vi "ICM Test Program.vi"() -> ()   [LabVIEW 2018]
doc: "Test Program.vi\n\nThis is a simple program that uses the ICM to demonstrate its structure.\n\nInstrument Communication Module Version 1.0\nDecember, 2017 Original Code Consulting David Thomson\n www.originalcode.com"
uses:
  Scaling/Scaling.lvclass
  Scaling/Scaling.lvclass/Scaling.ctl
  Query/Query.lvclass/Query.ctl
  Query/Read Cycle Time (ms).vi
  Initialize/Initialize.lvclass
  Parser/Parser.lvclass
  Output/Output.lvclass
  Query/Query.lvclass
  Bus/Bus.lvclass
panel:
  in  "Controller Values":dbl[](array[numeric])
  out "Enabled Controllers":string[](array[string])
  out "Scaled Values":dbl[](array[numeric])
  in  "stop":bool
  out "Enabled Channels":string[](array[string])
  out "Data Values":dbl[](array[numeric])
  out "String Read":string
  out "error out":errorcluster
  out "Config File":path
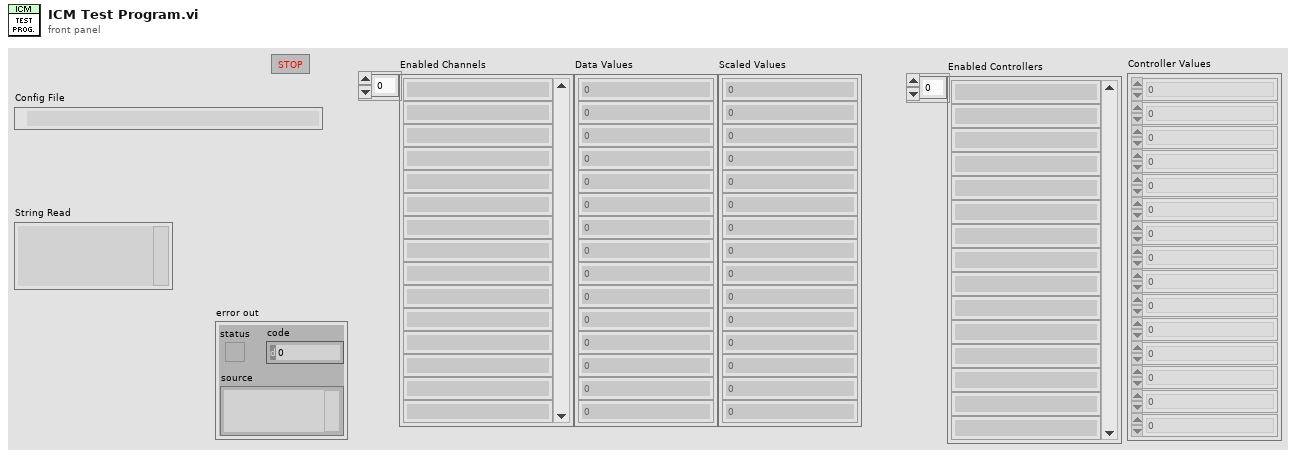
[diagram p1: front panel]
types:
  T1 = cluster{"Scaling Classes":refnum<class "Scaling.lvclass">[], "Scaling in":refnum<class "Scaling.lvclass">, "Used Scalings":string[], "Channel Names":string[]}
  T2 = typedef "Scaling Def.ctl" = cluster{"Channel":string, "Scaling":string, "Instance":string}
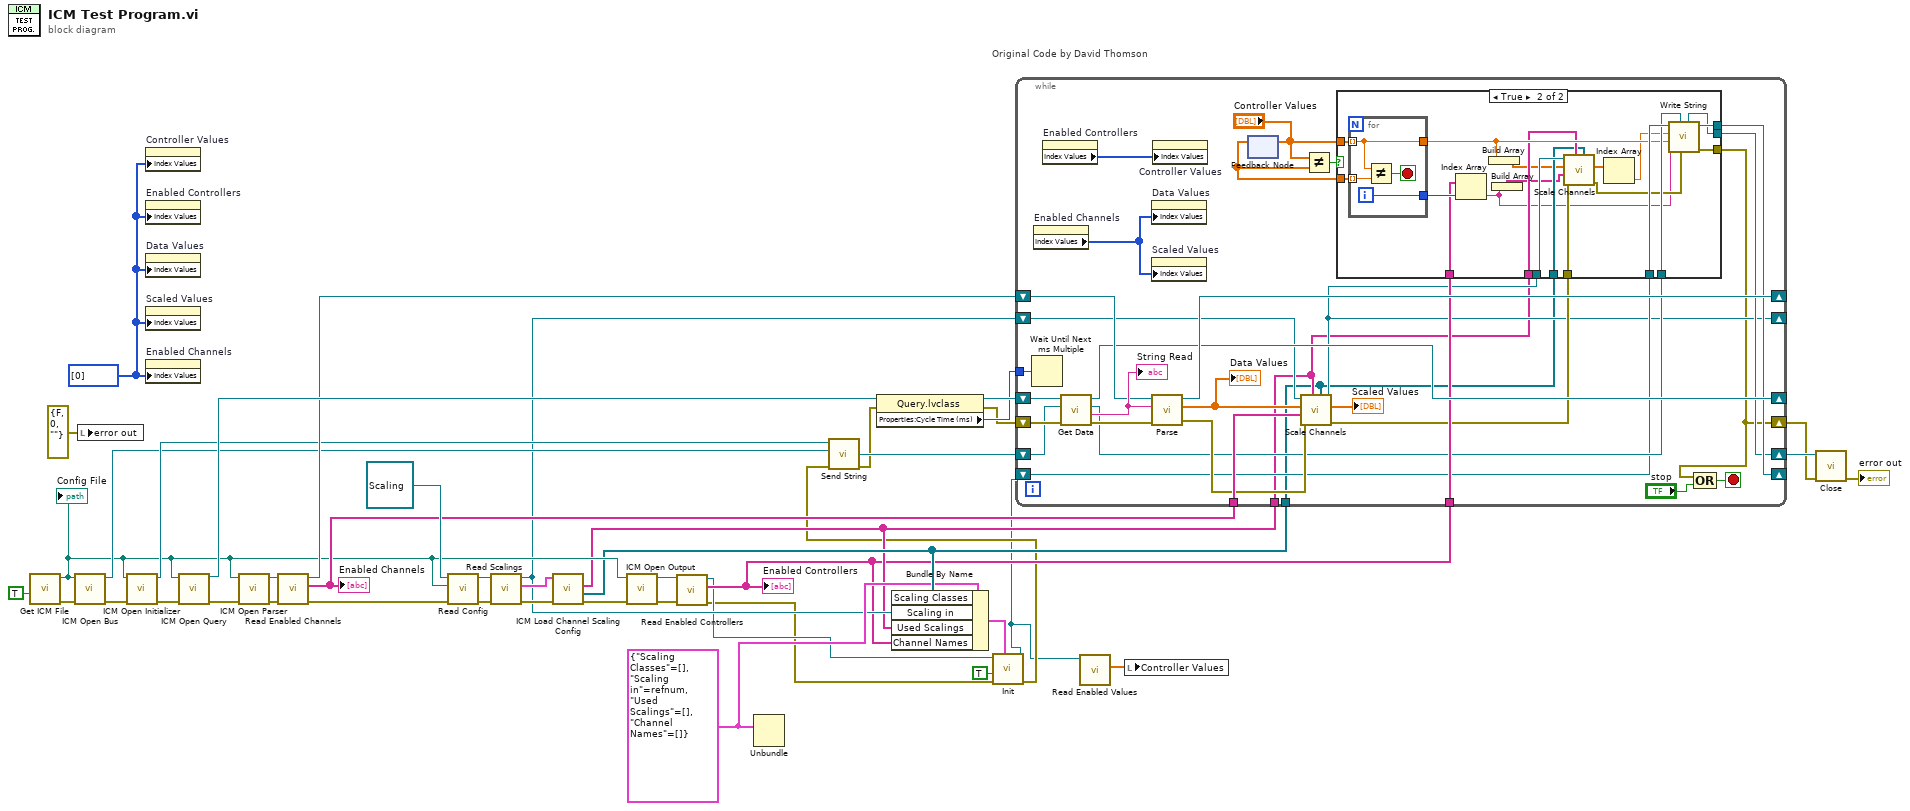
[diagram p0: block diagram]
diagram:
  w11 = T1 {"Scaling Classes"=[], "Scaling in"=refnum, "Used Scalings"=[], "Channel Names"=[]} ("Cluster")
  w13 = u32[] [0] ("Index Values")
  n1 = call "Get ICM File.vi"("Re-Init?"=TRUE) -> ("error out"=w37:errorcluster, "ICM File"=w16:path)  [unwired: 9 in]
  "Config File" <- w16
  n2 = call "ICM Open Bus.vi"("error in (no error)"=w37, "ICM File In"=w16) -> ("error out"=w23:errorcluster, "Bus out"=w21:refnum<class "Bus.lvclass">)  [unwired: 8 in]
  n3 = local write "error out"(errorcluster {"status"=FALSE, "code"=0, "source"=""} ("error out")) -> ()
  n4 = call "ICM Open Initializer.vi"("error in (no error)"=w23, "ICM File In"=w16) -> ("error out"=w14:errorcluster, "Init out"=w22:refnum<class "Initialize.lvclass">)  [unwired: 8 in]
  n5 = property on="Controller Values" class="Arr (strict)"("Index Values"=w13) -> ()  [unwired: 2 in, 2 out]
  n6 = property on="Enabled Controllers" class="Arr (strict)"("Index Values"=w13) -> ()  [unwired: 2 in, 2 out]
  n7 = property on="Data Values" class="Arr (strict)"("Index Values"=w13) -> ()  [unwired: 2 in, 2 out]
  n8 = property on="Scaled Values" class="Arr (strict)"("Index Values"=w13) -> ()  [unwired: 2 in, 2 out]
  n9 = property on="Enabled Channels" class="Arr (strict)"("Index Values"=w13) -> ()  [unwired: 2 in, 2 out]
  n10 = call "ICM Open Query.vi"("error in (no error)"=w14, "ICM File In"=w16) -> ("error out"=w38:errorcluster, "Query out"=w29:refnum<class "Query.lvclass">)  [unwired: 8 in]
  n11 = call "ICM Open Parser.vi"("error in (no error)"=w38, "ICM File In"=w16) -> ("error out"=w39:errorcluster, "Parser out"=w40:refnum<class "Parser.lvclass">)  [unwired: 8 in]
  n12 = call-dynamic "Read Enabled Channels.vi"("error in (no error)"=w39, "Parser in"=w40) -> ("error out"=w36:errorcluster, "Enabled Channels"=w34:string[], "Parser out"=w24:refnum<class "Parser.lvclass">)  [unwired: 7 in]
  "Enabled Channels" <- w34
  n13 = call-dynamic "Read Config.vi"("error in (no error)"=w36, "ICM File In"=w16, "Scaling in"=refnum<class "Scaling.lvclass"> refnum) -> ("error out"=w33:errorcluster, "Scaling out"=w31:refnum<class "Scaling.lvclass">)  [unwired: 7 in]
  n14 = call "Read Scalings.vi"("error in (no error)"=w33, "Scaling in"=w31) -> ("error out"=w32:errorcluster, "Scalings"=w30:T2[], "Scaling out"=w10:refnum<class "Scaling.lvclass">)  [unwired: 7 in]
  n15 = call "ICM Load Channel Scaling Config.vi"("error in (no error)"=w32, "Scalings"=w30) -> ("error out"=w18:errorcluster, "Scaling Classes"=w12:refnum<class "Scaling.lvclass">[], "Used Scalings"=w9:string[])  [unwired: 6 in, 1 out]
  n16 = call "ICM Open Output.vi"("error in (no error)"=w18, "ICM File In"=w16) -> ("error out"=w17:errorcluster, "Output out"=w15:refnum<class "Output.lvclass">)  [unwired: 8 in]
  n17 = call-dynamic "Read Enabled Controllers.vi"("error in (no error)"=w17, "Output in"=w15) -> ("error out"=w5:errorcluster, "Enabled Channels"=w8:string[], "Output out"=w6:refnum<class "Output.lvclass">)  [unwired: 7 in]
  "Enabled Controllers" <- w8
  n18 = Unbundle(w11) -> ()  [unwired: 4 out]
  n19 = Bundle By Name(cluster=w11, "Scaling Classes"=w12, "Scaling in"=w10, "Used Scalings"=w9, "Channel Names"=w8) -> (w7:T1)
  n20 = call-dynamic "Init.vi"("Cluster"=w7, "error in (no error)"=w5, "Init or Array"=TRUE, "Output in"=w6) -> ("error out"=w4:errorcluster, "Output out"=w2:refnum<class "Output.lvclass">)  [unwired: 6 in]
  n21 = call-dynamic "Send String.vi"("error in (no error)"=w4, "Bus In"=w21, "Init in"=w22) -> ("error out"=w19:errorcluster, "Bus Out"=w20:refnum<class "Bus.lvclass">)  [unwired: 4 in, 1 out]
  n22 = property class="Query.lvclass"(reference=w29, error in=w19) -> (reference out=w28:refnum<class "Query.lvclass">, error out=w26:errorcluster, "Properties:Cycle Time (ms)"=w27:u32)
  n23 = while "Original Code by David Thomson" {
    shift-right: [w45] -> w42
    shift-left: w26 -> [w73]
    tunnel: w27 -> [w69]
    tunnel: w34 -> [w66]
    tunnel: w9 -> [w47]
    tunnel: w12 -> [w46]
    shift-right: [w50] -> w43
    shift-left: w20 -> [w68]
    shift-right: [w63] -> _
    shift-left: w24 -> [w64]
    shift-right: [w62] -> _
    shift-left: w28 -> [w74]
    shift-right: [w48] -> _
    shift-left: w10 -> [w61]
    shift-right: [w51] -> _
    shift-left: w2 -> [w52]
    tunnel: w8 -> [w54]
    stop <- w71 stop-if-true
    n24 = Wait Until Next ms Multiple(millisecond multiple=w69) -> ()  [unwired: 1 out]
    n25 = property on="Enabled Channels" class="Arr (strict)"() -> ("Index Values"=w59:u32[])  [unwired: 2 in, 2 out]
    n26 = property on="Enabled Controllers" class="Arr (strict)"() -> ("Index Values"=w58:u32[])  [unwired: 2 in, 2 out]
    n27 = call-dynamic "Get Data.vi"("error in (no error)"=w73, "Bus In"=w68, "Query in"=w74) -> ("error out"=w72:errorcluster, "String Read"=w75:string, "Bus Out"=w53:refnum<class "Bus.lvclass">, "Query out"=w62:refnum<class "Query.lvclass">)  [unwired: 5 in]
    "String Read" <- w75
    n28 = property on="Data Values" class="Arr (strict)"("Index Values"=w59) -> ()  [unwired: 2 in, 2 out]
    n29 = property on="Scaled Values" class="Arr (strict)"("Index Values"=w59) -> ()  [unwired: 2 in, 2 out]
    n30 = call-dynamic "Parse.vi"("error in (no error)"=w72, "Data String"=w75, "Parser in"=w64) -> ("error out"=w60:errorcluster, "Data Values"=w67:dbl[], "Parser out"=w63:refnum<class "Parser.lvclass">)  [unwired: 6 in]
    "Data Values" <- w67
    n31 = property on="Controller Values" class="Arr (strict)"("Index Values"=w58) -> ()  [unwired: 2 in, 2 out]
    n32 = feedback-in #1("Controller Values") -> ()
    n33 = feedback #1() -> (w55:dbl[])  [unwired: 1 in]
    n34 = call "Scale Channels.vi"("Scaling Classes"=w46, "Used Scalings"=w47, "error in (no error)"=w60, "Channel Names"=w66, "Values In"=w67, "Scaling in"=w61) -> ("error out"=w49:errorcluster, "Values Out"=→"Scaled Values":dbl[], "Scaling out"=w48:refnum<class "Scaling.lvclass">)  [unwired: 3 in]
    n35 = Not Equal?(x="Controller Values", y=w55) -> (x != y?=w57:bool)
    n36 = case shown="True" w57 {
      tunnel: "Controller Values" -> [_ w98]
      tunnel: w55 -> [_ w97]
      tunnel: w54 -> [_ w95]
      tunnel: w53 -> [w77 w90]
      tunnel: w52 -> [w78 w94]
      tunnel: [w78 w93] -> w51
      tunnel: [w77 w91] -> w50
      tunnel: w49 -> [w76 w86]
      tunnel: [w76 w92] -> w45
      tunnel: w48 -> [_ w88]
      tunnel: w47 -> [_ w84]
      tunnel: w46 -> [_ w83]
      frame False {
      }
      frame True {
        n37 = for {
          tunnel: w98 -> [w100] mode=indexing
          tunnel: w97 -> [w102] mode=indexing
          tunnel: [w100] -> w89
          tunnel: [w99] -> w96
          i -> [w99]
          stop <- w101 stop-if-true
          n38 = Not Equal?(x=w100, y=w102) -> (x != y?=w101:bool)
        }
        n39 = Index Array(array=w95, index=w96) -> (element=w79:string)
        n40 = Build Array(w89) -> (w82:dbl[])
        n41 = Build Array(w79) -> (w81:string[])
        n42 = call "Scale Channels.vi"("Scaling Classes"=w83, "Used Scalings"=w84, "error in (no error)"=w86, "Channel Names"=w81, "Values In"=w82, "Scaling in"=w88) -> ("error out"=w87:errorcluster, "Values Out"=w85:dbl[])  [unwired: 3 in, 1 out]
        n43 = Index Array(array=w85) -> (element=w80:dbl)  [unwired: 1 in]
        n44 = call-dynamic "Write String.vi"("error in (no error)"=w87, "Bus In"=w90, "Channel Name"=w79, "Data Value Engineering"=w89, "Data Value Native"=w80, "Output in"=w94) -> ("error out"=w92:errorcluster, "Output out"=w93:refnum<class "Output.lvclass">, "Bus Out"=w91:refnum<class "Bus.lvclass">)  [unwired: 3 in]
      }
    }
    n45 = Compound Arithmetic op=OR(w45, "stop") -> (w71:bool)
  }
  n46 = call-dynamic "Read Enabled Values.vi"("Output in"=w2) -> ("Data Values Engineering"=w1:dbl[])  [unwired: 7 in, 3 out]
  n47 = local write "Controller Values"(w1) -> ()
  n48 = call-dynamic "Close.vi"("error in (no error)"=w42, "Bus in"=w43) -> ("error out"=→"error out":errorcluster)  [unwired: 8 in, 1 out]
